vi "testDataPass_v3,0_host.vi"() -> ()   [LabVIEW 2014]
panel:
  out "error out 2":errorcluster
  out "error out":errorcluster
  in  "stop":bool
  out "data out":u16
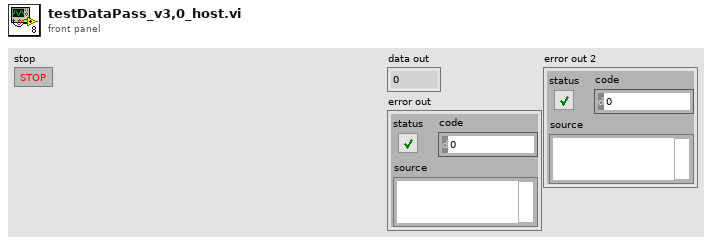
[diagram p1: front panel]
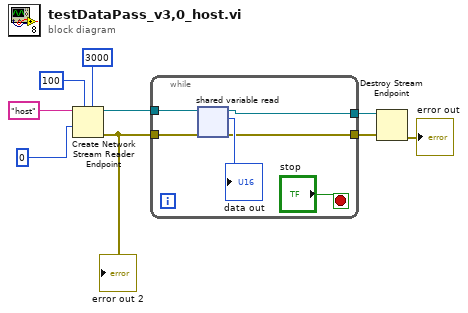
[diagram p0: block diagram]
diagram:
  n1 = Create Network Stream Reader Endpoint(5:3000 ("timeout in ms (-1)"), 7:100 ("reader buffer size"), 9:u16 0, 11:"host" ("reader name")) -> (0:w6:errorcluster, 3:w7:refnum<k21>)  [unwired: 3 in]
  "error out 2" <- w6
  n2 = while {
    tunnel: w7 -> [w15]
    tunnel: w6 -> [w14]
    tunnel: [w11] -> w5
    tunnel: [w10] -> w4
    stop <- "stop" stop-if-true
    n3 = shared-variable-read(w15, w14) -> (w11:refnum<k21>, w10:errorcluster, →"data out":u16)  [unwired: 1 in, 1 out]
  }
  n4 = Destroy Stream Endpoint(8:w4, 11:w5) -> (0:→"error out":errorcluster)
